vi "WPI_ADIS16448RunLoop.vi"(8 "error in":errorcluster, 11 "ADIS16448DevRef in":T2 {"Registers to Read" items=["XGYRO_OUT"=4, "YGYRO_OUT"=6, "ZGYRO_OUT"=8, "XACCL_OUT"=10, "YACCL_OUT"=12, "ZACCL_OUT"=14, "XMAGN_OUT"=16, "YMAGN_OUT"=18, "ZMAGN_OUT"=20, "BARO_OUT"=22, "TEMP_OUT"=24]}) -> (0 "error out":errorcluster, 3 "ADIS16448DevRef out":T2 {"Registers to Read" items=["XGYRO_OUT"=4, "YGYRO_OUT"=6, "ZGYRO_OUT"=8, "XACCL_OUT"=10, "YACCL_OUT"=12, "ZACCL_OUT"=14, "XMAGN_OUT"=16, "YMAGN_OUT"=18, "ZMAGN_OUT"=20, "BARO_OUT"=22, "TEMP_OUT"=24]})   [LabVIEW 2014, in "ADIS16448.lvlib"]
uses:
  ADIS16448.lvlib
  Typedef/WPI_ADIS16448Ref.ctl
  <vilib>/Rock Robotics/WPI/SPI/WPI_SPIDevRef.ctl
  <vilib>/Rock Robotics/SystemInterfaces/Typedef/FPGA_TypedefDigitalModule.ctl
  <vilib>/Rock Robotics/SystemInterfaces/spilib/spi_bus.ctl
  <vilib>/Rock Robotics/SystemInterfaces/CounterEncoderSourceConvertion/FPGA_CounterEncoderSourceConvertionLVSourceType.ctl
  <vilib>/Rock Robotics/SystemInterfaces/DIO/FPGA_DIODigitalSourceChannel.ctl
  <vilib>/Rock Robotics/SystemInterfaces/AnalogTrigger/FPGA_AnalogTriggerIndex.ctl
  <vilib>/Rock Robotics/SystemInterfaces/AnalogTrigger/FPGA_AnalogTriggerOutType.ctl
  Typedef/WPI_ADIS16448SampleMode.ctl
  Typedef/WPI_ADIS16448DataRegisters.ctl
  Typedef/WPI_ADIS16448ReadingsDVR.ctl
  Typedef/WPI_ADIS16448Readings.ctl
  <vilib>/Rock Robotics/SystemInterfaces/Interrupt/FPGA_InterruptRef.ctl
  <vilib>/Rock Robotics/SystemInterfaces/Interrupt/FPGA_InterruptIndex.ctl
  <vilib>/Rock Robotics/SystemInterfaces/Utilities/FPGA_UtilitiesRead LocalTime.vi
panel:
  out "Ring":T1=4 items=["XGYRO_OUT"=4, "YGYRO_OUT"=6, "ZGYRO_OUT"=8, "XACCL_OUT"=10, "YACCL_OUT"=12, "ZACCL_OUT"=14, "XMAGN_OUT"=16, "YMAGN_OUT"=18, "ZMAGN_OUT"=20, "BARO_OUT"=22, "TEMP_OUT"=24]
  out "Gyro Angle":dbl
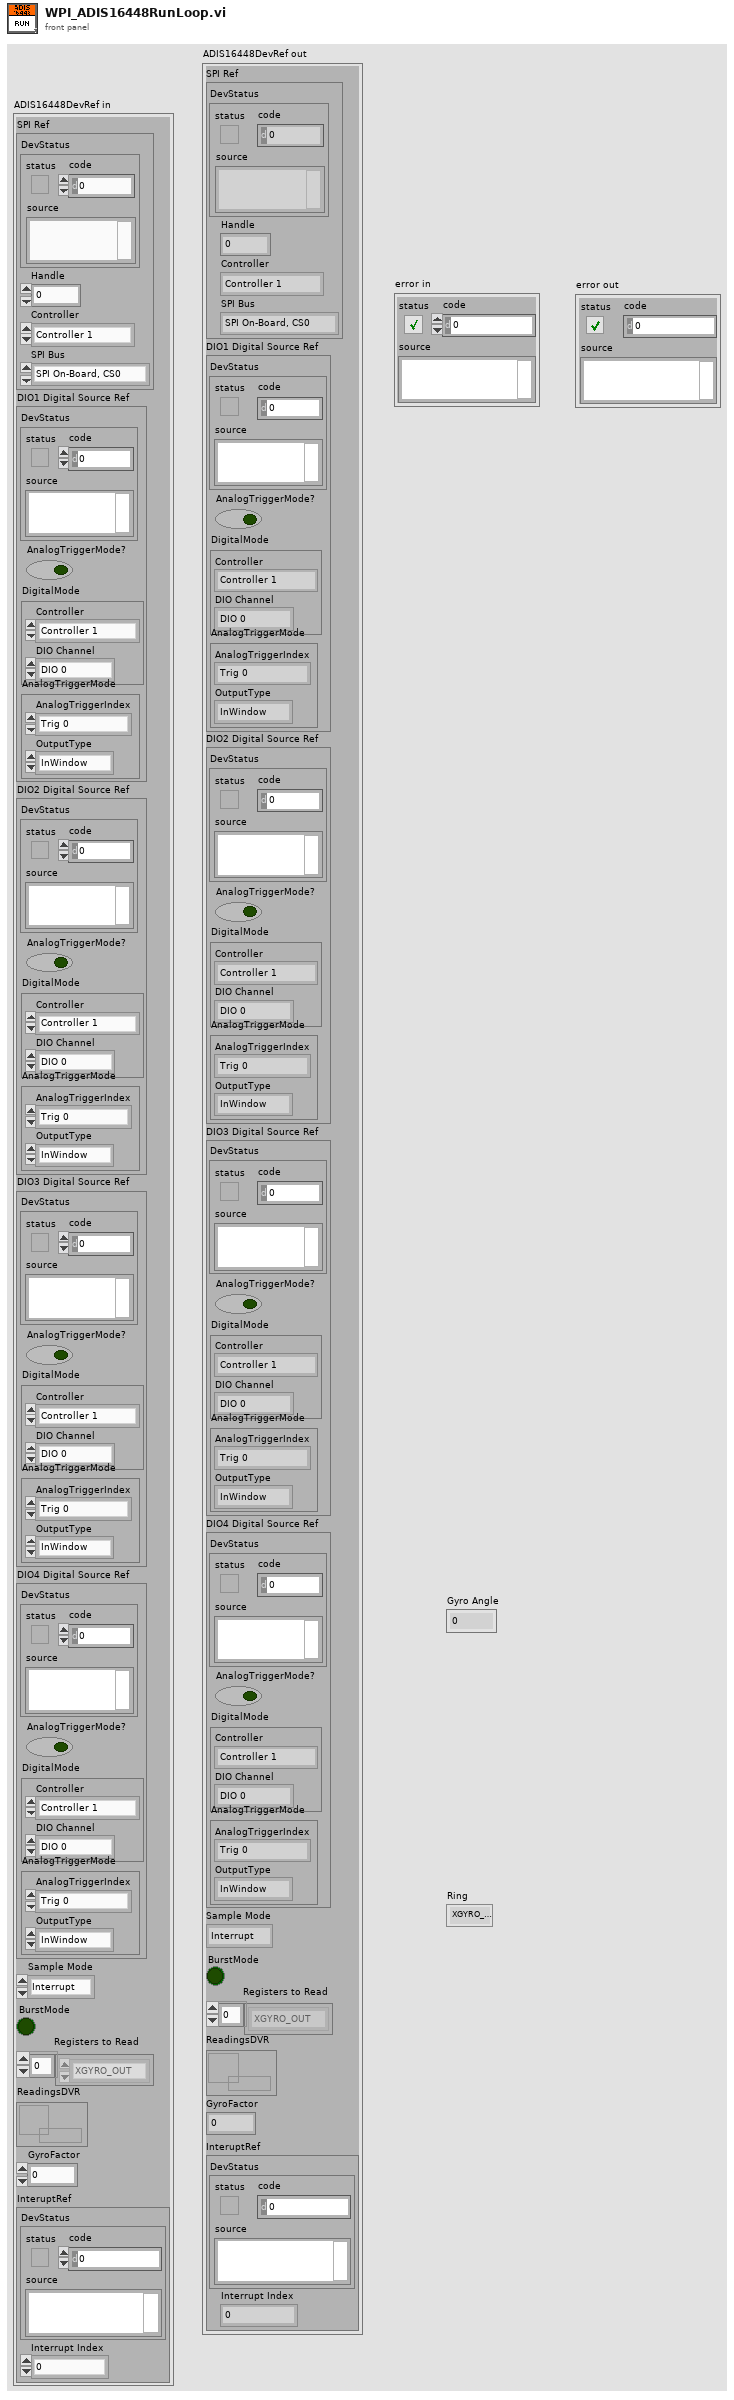
[diagram p1: front panel]
types:
  T1 = typedef "ADIS16448.lvlib/WPI_ADIS16448DataRegisters.ctl" = u16
  T2 = typedef "ADIS16448.lvlib/WPI_ADIS16448Ref.ctl" = cluster{"SPI Ref":T3, "DIO1 Digital Source Ref":T6, "DIO2 Digital Source Ref":T6, "DIO3 Digital Source Ref":T6, "DIO4 Digital Source Ref":T6, "Sample Mode":T10, "BurstMode":bool, "Registers to Read":T1[], "ReadingsDVR":T11, "GyroFactor":dbl, "InteruptRef":T12}
  T3 = typedef "WPI_SPIDevRef.ctl" = cluster{"DevStatus":errorcluster, "Handle":i32, "Controller":T4, "SPI Bus":T5}
  T4 = typedef "FPGA_TypedefDigitalModule.ctl" = enum16{"Controller 1"}
  T5 = typedef "spi_bus.ctl" = enum16{"SPI On-Board, CS0", "SPI On-Board, CS1", "SPI On-Board, CS2", "SPI On-Board, CS3", "SPI MXP", "Invalid"}
  T6 = typedef "FPGA_CounterEncoderSourceConvertionLVSourceType.ctl" = cluster{"DevStatus":errorcluster, "AnalogTriggerMode?":bool, "DigitalMode":cluster{"Controller":T4, "DIO Channel":T7}, "AnalogTriggerMode":cluster{"AnalogTriggerIndex":T8, "OutputType":T9}}
  T7 = typedef "FPGA_DIODigitalSourceChannel.ctl" = enum8{"DIO 0", "DIO 1", "DIO 2", "DIO 3", "DIO 4", "DIO 5", "DIO 6", "DIO 7", "DIO 8", "DIO 9", "DIO MXP 0", "DIO MXP 1", "DIO MXP 2", "DIO MXP 3", "DIO MXP 4", "DIO MXP 5", "DIO MXP 6", "DIO MXP 7", "DIO MXP 8", "DIO MXP 9", "DIO MXP 10", "DIO MXP 11", "DIO MXP 12", "DIO MXP 13", "DIO MXP 14", "DIO MXP 15", "Disabled"}
  T8 = typedef "FPGA_AnalogTriggerIndex.ctl" = enum8{"Trig 0", "Trig 1", "Trig 2", "Trig 3", "Trig 4", "Trig 5", "Trig 6", "Trig 7", "Invalid"}
  T9 = typedef "FPGA_AnalogTriggerOutType.ctl" = enum16{"InWindow", "TriggerState", "Rising", "Falling"}
  T10 = typedef "ADIS16448.lvlib/WPI_ADIS16448SampleMode.ctl" = enum16{"Interrupt", "Polled"}
  T11 = typedef "ADIS16448.lvlib/WPI_ADIS16448ReadingsDVR.ctl" = refnum<data-value>
  T12 = typedef "FPGA_InterruptRef.ctl" = cluster{"DevStatus":errorcluster, "Interrupt Index":T13}
  T13 = typedef "FPGA_InterruptIndex.ctl" = enum8{"0", "1", "2", "3", "4", "5", "6", "7", "Invalid"}
  T14 = typedef "ADIS16448.lvlib/WPI_ADIS16448Readings.ctl" = u16[]
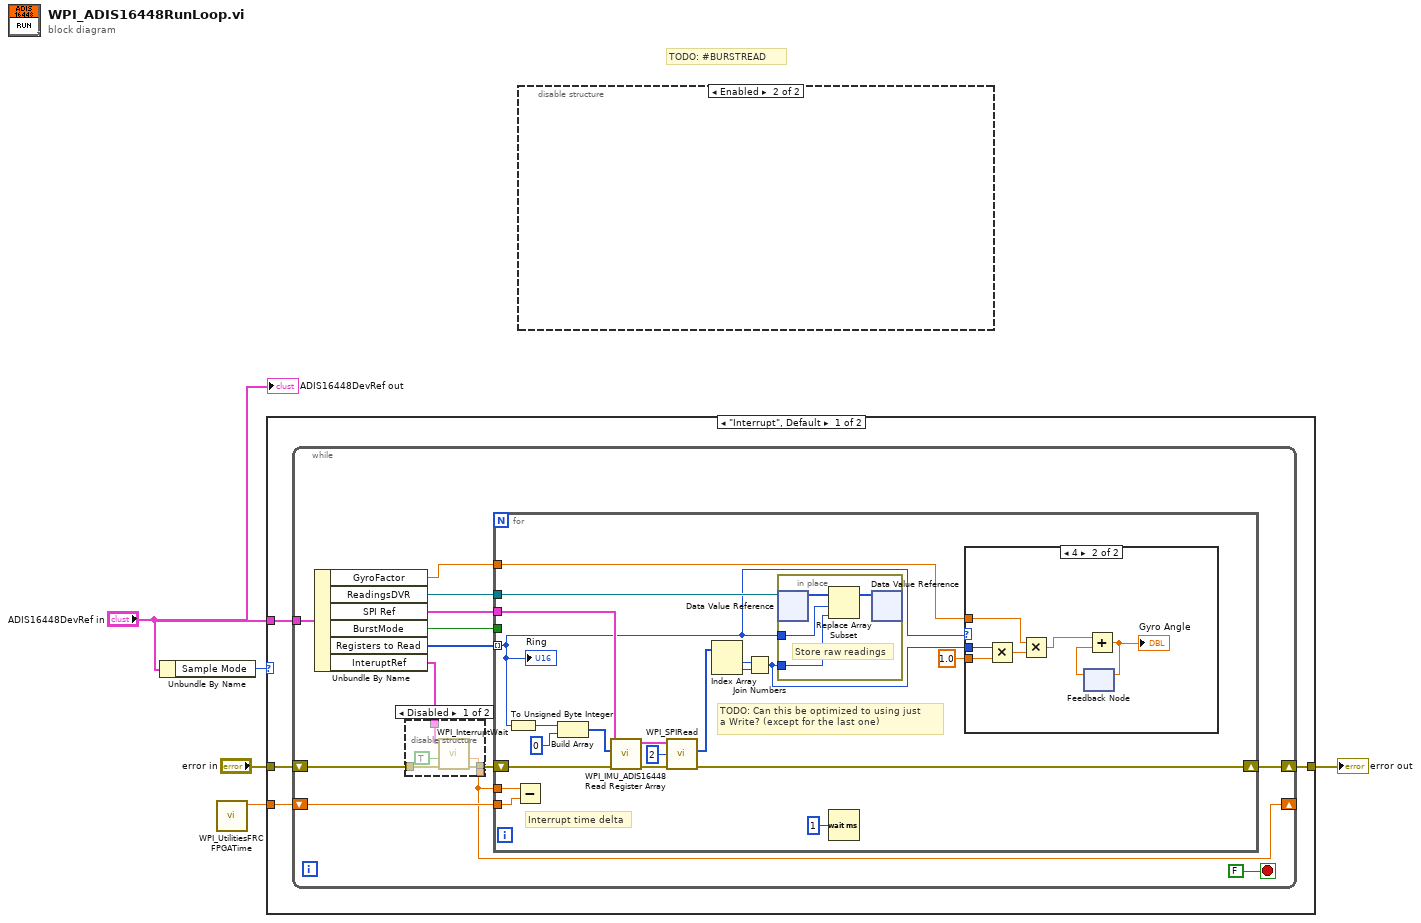
[diagram p0: block diagram]
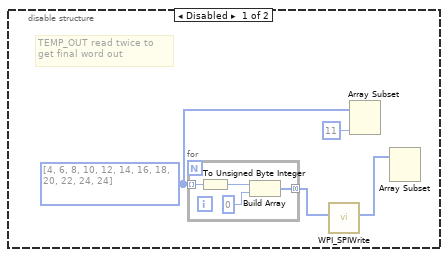
[diagram p2: hidden frame]
diagram:
  # "TODO: #BURSTREAD"
  n1 = Unbundle By Name("ADIS16448DevRef in") -> ("Sample Mode"=w2:T10)
  n2 = call <vilib>:"WPI_UtilitiesFRC FPGATime.vi"() -> ("FPGA Time"=w1:dbl)  [unwired: 10 in, 1 out]
  n3 = case shown="\"Interrupt\", Default" w2 {
    tunnel: "ADIS16448DevRef in" -> [w9 _]
    tunnel: "error in" -> [w8 w59]
    tunnel: [w7 w59] -> w4
    tunnel: w1 -> [w6 _]
    frame "Interrupt", Default {
      n4 = while {
        tunnel: w9 -> [w22]
        shift-right: [w17] -> w7
        shift-left: w8 -> [w21]
        shift-right: [w12] -> _
        shift-left: w6 -> [w13]
        stop <- FALSE stop-if-true
        n5 = Unbundle By Name(w22) -> ("GyroFactor"=w11:dbl, "ReadingsDVR"=w19:T11, "SPI Ref"=w14:T3, "BurstMode"=w15:bool, "Registers to Read"=w16:T1[], "InteruptRef"=w10:T12)
        n6 = disable-structure shown="Disabled" {
          disable-tunnel: w21 -> [w27 _]
          disable-tunnel: [w26 _] -> w18
          disable-tunnel: [w25 _] -> w12
          disable-tunnel: w10 -> [w23 _]
          frame Disabled {
            n7 = call <vilib>:"WPI_InterruptWait.vi"("error in (no error)"=w27, "Ignore Previous Interrupts"=TRUE, "InteruptRef"=w23) -> ("error out"=w26:errorcluster, "TimeStamp"=w25:dbl)  [unwired: 4 in, 3 out]
          }
          frame Enabled {
          }
        }
        n8 = for {
          tunnel: w19 -> [w44]
          shift-right: [w46] -> w17
          shift-left: w18 -> [w47]
          tunnel: w16 -> [w30] mode=indexing
          tunnel: w15 -> [_]
          tunnel: w14 -> [w45]
          tunnel: w12 -> [w34]
          tunnel: w13 -> [w33]
          tunnel: w11 -> [w31]
          # "Interrupt time delta"
          # "TODO: Can this be optimized to using just\na Write? (except for the last one)"
          n9 = To Unsigned Byte Integer(number=w30) -> (unsigned 8bit integer=w38:u8)
          n10 = Subtract(x=w34, y=w33) -> ()  [unwired: 1 out]
          n11 = Build Array(w38, u8 0) -> (w40:u8[])
          n12 = call "WPI_IMU_ADIS16448 Read Register Array.vi"("error in"=w47, "Registers"=w40, "SPI Ref"=w45) -> ("error out"=w43:errorcluster, "SPIDevRef"=w42:T3)  [unwired: 6 in, 1 out]
          n13 = call <vilib>:"WPI_SPIRead.vi"("error in (no error)"=w43, "Num to Read"=2, "SPIDevRef"=w42) -> ("error out"=w46:errorcluster, "Received Data"=w37:u8[])  [unwired: 6 in, 1 out]
          n14 = Index Array(array=w37) -> (element #1=w36:u8, element #2=w35:u8)  [unwired: 2 in]
          n15 = Join Numbers(hi=w36, lo=w35) -> ((hi.lo)=w32:u16)
          n16 = in-place {
            in-place-border: w32 -> [w58]
            in-place-border: w30 -> [w55]
            # "Store raw readings"
            n17 = in-place-dvr #1(w44) -> (w57:T14)  [unwired: 1 out]
            n18 = Replace Array Subset(array=w57, new element=w58, index=w55) -> (w56:T14)
            n19 = in-place-dvr #1(w56) -> ()  [unwired: 2 out]
          }
          n20 = Wait (ms)(milliseconds to wait=u32 1) -> ()  [unwired: 1 out]
          n21 = case shown="4" w30 {
            tunnel: 1.0 -> [_ w53]
            tunnel: w32 -> [_ w54]
            tunnel: w31 -> [_ w51]
            frame 0, Default {
            }
            frame 4 {
              n22 = Multiply(x=w54, y=w53) -> (x*y=w52:dbl)
              n23 = Multiply(x=w51, y=w52) -> (x*y=w50:dbl)
              n24 = feedback #2() -> (w48:dbl)  [unwired: 1 in]
              n25 = Add(x=w50, y=w48) -> (x+y=w49:dbl)
              "Gyro Angle" <- w49
              n26 = feedback-in #2(w49) -> ()
            }
          }
          "Ring" <- w30
        }
      }
    }
    frame "Polled" {
    }
  }
  "error out" <- w4
  n27 = disable-structure shown="Enabled" {
    frame Disabled {
      w63 = T1[] [4, 6, 8, 10, 12, 14, 16, 18, 20, 22, 24, 24] items=["XGYRO_OUT"=4, "YGYRO_OUT"=6, "ZGYRO_OUT"=8, "XACCL_OUT"=10, "YACCL_OUT"=12, "ZACCL_OUT"=14, "XMAGN_OUT"=16, "YMAGN_OUT"=18, "ZMAGN_OUT"=20, "BARO_OUT"=22, "TEMP_OUT"=24] ("Registers to Read")
      # "TEMP_OUT read twice to \nget final word out"
      n28 = for {
        tunnel: w63 -> [w69] mode=indexing
        tunnel: [w66] -> w62 mode=concatenating
        n29 = To Unsigned Byte Integer(number=w69) -> (unsigned 8bit integer=w67:u8)
        n30 = Build Array(w67, u8 0) -> (w66:u8[])
      }
      n31 = call <vilib>:"WPI_SPIWrite.vi"("Data To Send"=w62) -> ("Received Data"=w65:u8[], "error in (no error)"=w61:errorcluster, "SPIDevRef"=w60:T3)  [unwired: 6 in, 2 out]
      n32 = Array Subset(array=w63, length=11) -> ()  [unwired: 1 in, 1 out]
      n33 = Array Subset(array=w65) -> ()  [unwired: 2 in, 1 out]
    }
    frame Enabled {
    }
  }
  "ADIS16448DevRef out" <- "ADIS16448DevRef in"
